vi "Set IConfiguration.vi"(10 "IConfiguration":refnum<class "IConfiguration.lvclass">, 11 "PCAN Basic in":refnum<class "PCAN Basic Base Configure Strategy.lvclass">) -> (3 "PCAN Basic out":refnum<class "PCAN Basic Base Configure Strategy.lvclass">)   [LabVIEW 2025, in "PCAN Basic Base Configure Strategy.lvclass"]
uses:
  PCAN Basic Base Configure Strategy.lvclass
  Source/Interfaces/IConfiguration/IConfiguration.lvclass
  PCAN Basic Base Configure Strategy.lvclass/PCAN Basic Base Configure Strategy.ctl
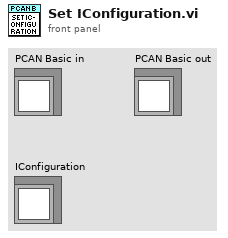
[diagram p1: front panel]
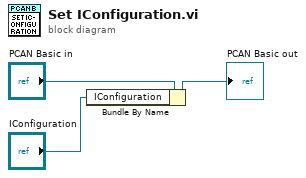
[diagram p0: block diagram]
diagram:
  n1 = Bundle By Name(cluster="PCAN Basic in", "IConfiguration"="IConfiguration") -> (→"PCAN Basic out":refnum<class "PCAN Basic Base Configure Strategy.lvclass">)
